vi "Set Output Impedance.vi"(8 "error in (no error)":errorcluster, 10 "Output Impedance (0: 50 ohm)":u32(ring) items=["50 ohm", "1 Mohm"], 11 "VISA resource name":refnum<visa-resource-name>) -> (0 "error out":errorcluster, 3 "VISA resource name out":refnum<visa-resource-name>)   [LabVIEW 2013, in "Fluke 5XXX Series Multicalibrators.lvlib"]
doc: "This VI programs the oscilloscope’s output impedance.\n\nNote:\n\nThis VI is available only for instrument models 5500A and 5520A with oscilloscope option SC300 (SC600 or SC1100)."
uses:
  Fluke 5XXX Series Multicalibrators.lvlib
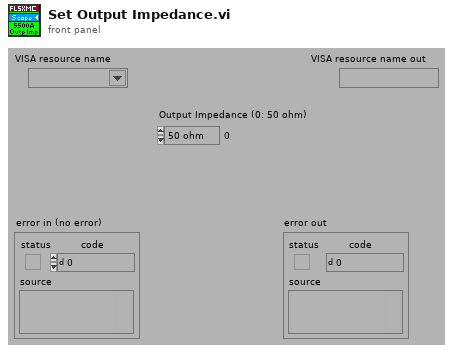
[diagram p1: front panel]
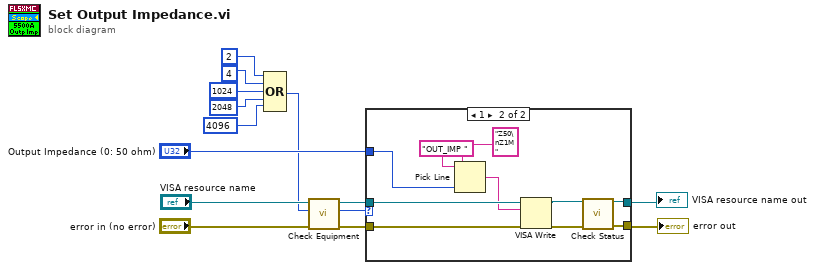
[diagram p0: block diagram]
diagram:
  n1 = Compound Arithmetic op=OR(2 ("Numeric"), 4 ("Numeric"), 1024 ("Numeric"), 2048 ("Numeric"), 4096 ("Numeric")) -> (w3:i32)
  n2 = call "Check Equipment.vi"("error in (no error)"="error in (no error)", "Bit Mask"=w3, "VISA resource name"="VISA resource name") -> ("error out"=w9:errorcluster, "Present?"=w8:u32, "VISA resource name out"=w7:refnum<visa-resource-name>)  [unwired: 6 in]
  n3 = case shown="1" w8 {
    tunnel: "Output Impedance (0: 50 ohm)" -> [_ w21]
    tunnel: [w15 w17] -> w1
    tunnel: w9 -> [w16 w24]
    tunnel: w7 -> [w15 w23]
    tunnel: [w16 w20] -> w2
    frame 0, Default {
    }
    frame 1 {
      n4 = Pick Line(string ("")="OUT_IMP " ("Reset Command"), multi-line string="Z50\nZ1M", line index=w21) -> (output string=w22:string)
      n5 = VISA Write(VISA resource name=w23, write buffer=w22, error in (no error)=w24) -> (VISA resource name out=w18:refnum<visa-resource-name>, error out=w19:errorcluster)  [unwired: 1 out]
      n6 = call "Check Status.vi"("VISA resource name"=w18, "error in (no error)"=w19) -> ("VISA resource name out"=w17:refnum<visa-resource-name>, "error out"=w20:errorcluster)  [unwired: 12 in]
    }
  }
  "VISA resource name out" <- w1
  "error out" <- w2
